vi "Get Display Mode.vi"(8 "Error In":errorcluster, 11 "Display Manager In":refnum<class "Display Manager.lvclass">) -> (0 "Error Out":errorcluster, 2 "Display Mode":T1, 3 "Display Manager Out":refnum<class "Display Manager.lvclass">)   [LabVIEW 2019, in "Display Manager.lvclass"]
uses:
  Display Manager.lvclass
  Private/Controls/Display Mode.ctl
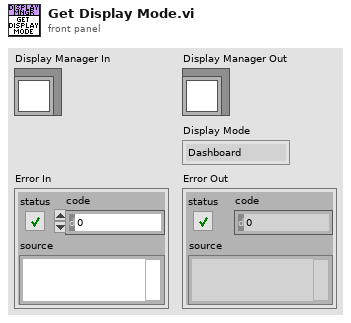
[diagram p1: front panel]
types:
  T1 = typedef "Display Manager.lvclass/Display Mode.ctl" = enum16{"Dashboard", "Audio Analyzer"}
  T2 = typedef "Display Manager.lvclass/Data.ctl" = cluster{"Display":refnum<class "Display.lvclass">, "Open Weather Session":refnum<class "Open Weather Session.lvclass">, "Display Mode":T1}
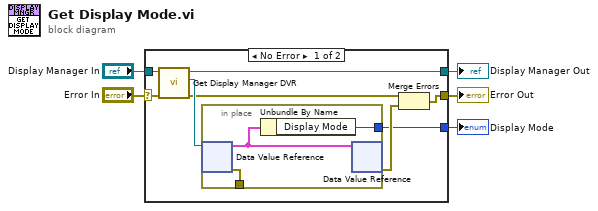
[diagram p0: block diagram]
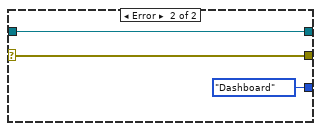
[diagram p2: hidden frame]
diagram:
  n1 = case shown="No Error" "Error In" {
    selector: "Error In" -> [w9 w18]
    tunnel: [w11 w18] -> w2
    tunnel: [w8 w19] -> w4
    tunnel: "Display Manager In" -> [w10 w19]
    tunnel: [w12 Display_Mode."Dashboard" ("Display Mode")] -> w1
    frame No Error {
      n2 = call "Get Display Manager DVR.vi"("Error In"=w9, "Display Manager In"=w10) -> ("Error Out"=w6:errorcluster, "DVR"=w7:refnum<data-value>, "Display Manager Out"=w8:refnum<class "Display Manager.lvclass">)  [unwired: 7 in]
      n3 = in-place {
        in-place-border: [w14] -> w12
        in-place-border: [w16] -> _
        n4 = in-place-dvr #1(w7) -> (w15:T2, w16:errorcluster)
        n5 = Unbundle By Name(w15) -> ("Display Mode"=w14:T1)
        n6 = in-place-dvr #1(w15) -> (w13:errorcluster)  [unwired: 1 out]
      }
      n7 = Merge Errors(w6, w13) -> (w11:errorcluster)
    }
    frame Error {
    }
  }
  "Display Manager Out" <- w4
  "Error Out" <- w2
  "Display Mode" <- w1
